vi "serialize.ob.cmd.vi"(11 "OrderBook.Commands.in":T1[](array[typedef])=[{"type"=enum."AddOrder", "side"=66, "orderId "=48, "quantity"=20000, "symbol"=4702127773838221344, "price"=9050, "executed.qty"=0, "canceled.qty"=0, "remaining.qty"=0, "seconds"=0, "nanoseconds"=0, "Add"=FALSE, "Edit"=FALSE, "Remove"=FALSE, "seq no"=0}] {"symbol" format="%.0x"; "orderId" format="%.0x"; "side" format="%.0x"}) -> (3 "Words.Out":u64[](array[numeric])=[1, 66, 48, 20000, 4702127773838221344, 9050, 0, 0, 0, 0, 0, 0, 0, 0, 0, 0, 2, 66, 48, 0, 0, 9050, 200, 0, 0, 0, 0, 0, 0, 0, 0, 0, 5, 66, 48, 1400, 6076284164848492576, 9050, 0, 0, 0, 0, 0, 0, 0, 0, 0, 0] format="%.0x")   [LabVIEW 2020, in "fpganow.common.host.lvlib"]
uses:
  fpganow.common.host.lvlib
  fpga/orderbook.command.ctl
  fpga/orderbook.command.type.ctl
  fpga/fpganow.common.fpga.lvlib
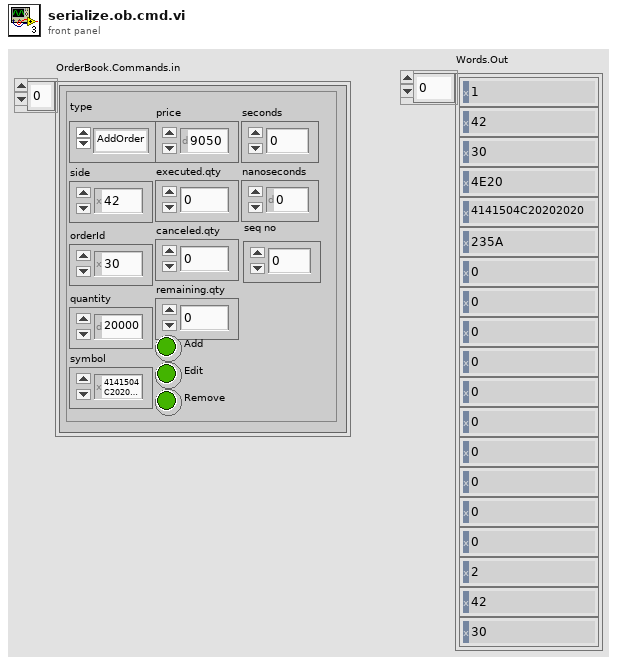
[diagram p1: front panel]
types:
  T1 = typedef "fpganow.common.fpga.lvlib/orderbook.command.ctl" = cluster{"type":T2, "side":u8, "orderId ":u64, "quantity":u32, "symbol":u64, "price":u64, "executed.qty":u32, "canceled.qty":u32, "remaining.qty":u32, "seconds":u64, "nanoseconds":u64, "Add":bool, "Edit":bool, "Remove":bool, "seq no":u32}
  T2 = typedef "fpganow.common.fpga.lvlib/orderbook.command.type.ctl" = enum8{"Time", "AddOrder", "OrderExecuted", "OrderExecutedAtPrice", "ReduceSize", "ModifyOrder", "DeleteOrder", "Get.Everything", "Get.All.Orders", "Get.Top"}
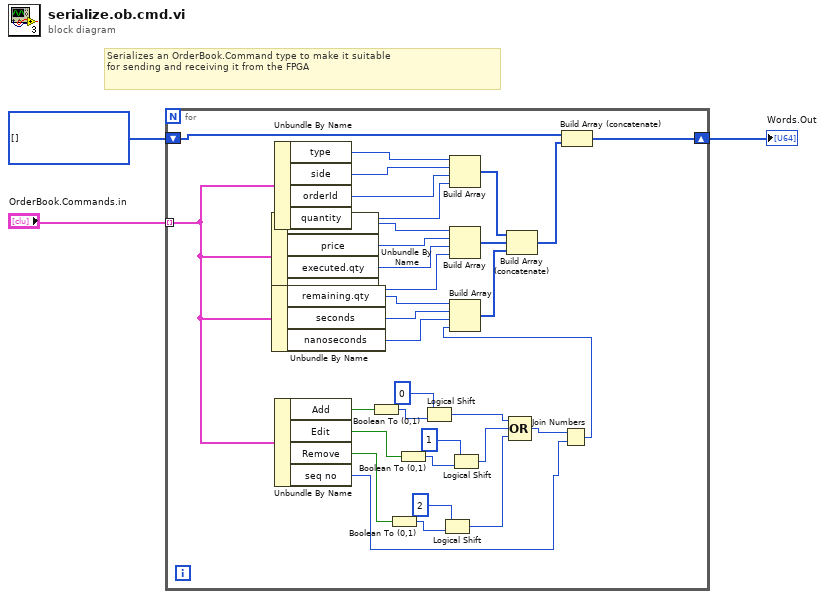
[diagram p0: block diagram]
diagram:
  # "Serializes an OrderBook.Command type to make it suitable\nfor sending and receiving it from the FPGA"
  n1 = for {
    tunnel: "OrderBook.Commands.in" -> [w23] mode=indexing
    shift-right: [w25] -> w1
    shift-left: u64[] [] -> [w27]
    n2 = Unbundle By Name(w23) -> ("symbol"=w36:u64, "price"=w35:u64, "executed.qty"=w34:u32, "canceled.qty"=w33:u32)
    n3 = Unbundle By Name(w23) -> ("remaining.qty"=w32:u32, "seconds"=w31:u64, "nanoseconds"=w24:u64)
    n4 = Unbundle By Name(w23) -> ("type"=w22:T2, "side"=w21:u8, "orderId"=w20:u64, "quantity"=w19:u32)
    n5 = Unbundle By Name(w23) -> ("Add"=w18:bool, "Edit"=w8:bool, "Remove"=w9:bool, "seq no"=w12:u32)
    n6 = Boolean To (0,1)(Boolean=w18) -> (0, 1=w16:i16)
    n7 = Boolean To (0,1)(Boolean=w9) -> (0, 1=w11:i16)
    n8 = Boolean To (0,1)(Boolean=w8) -> (0, 1=w14:i16)
    n9 = Logical Shift(y=u32 0, x=w16) -> (x << y=w5:i16)
    n10 = Logical Shift(y=u32 2, x=w11) -> (x << y=w7:i16)
    n11 = Build Array(w22, w21, w20, w19) -> (w30:u64[])
    n12 = Build Array(w36, w35, w34, w33) -> (w29:u64[])
    n13 = Logical Shift(y=u32 1, x=w14) -> (x << y=w6:i16)
    n14 = Compound Arithmetic op=OR(w5, w6, w7) -> (w4:i16)
    n15 = Join Numbers(hi=w4, lo=w12) -> ((hi.lo)=w17:u64)
    n16 = Build Array(w32, w31, w24, w17) -> (w28:u64[])
    n17 = Build Array (concatenate)(w30, w29, w28) -> (w26:u64[])
    n18 = Build Array (concatenate)(w27, w26) -> (w25:u64[])
  }
  "Words.Out" <- w1
